vi "Focus Move Absolute.vi"(8 "error in (no error)":errorcluster, 9 "Position":i32, 10 "Motor (0:n-1)":i32, 11 "NewFocus in":refnum<class "NewFocus.lvclass">) -> (0 "error out":errorcluster, 3 "NewFocus out":refnum<class "NewFocus.lvclass">)   [LabVIEW 2021, in "NewFocus.lvclass"]
uses:
  NewFocus.lvclass
  NewFocus.lvclass/NewFocus.ctl
  Focus Class/Focus Class.lvclass
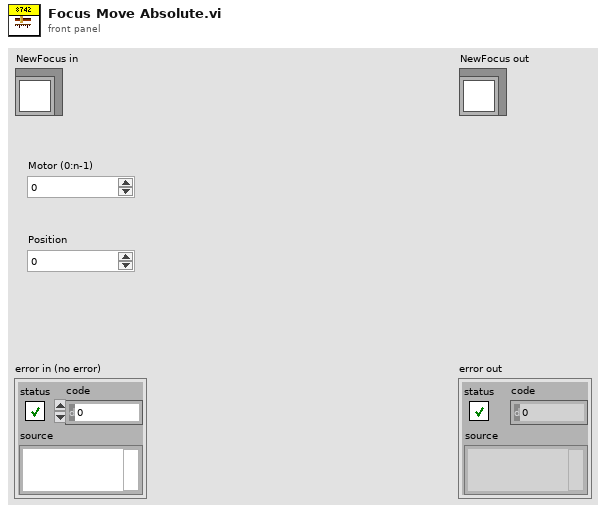
[diagram p1: front panel]
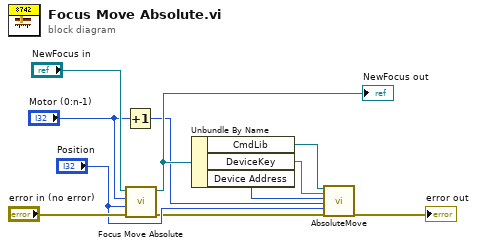
[diagram p0: block diagram]
diagram:
  n1 = Increment(x="Motor (0:n-1)") -> (x+1=w1:i32)
  n2 = call-parent "Focus Move Absolute.vi"("error in (no error)"="error in (no error)", "Position"="Position", "Motor (0:n-1)"="Motor (0:n-1)", "Focus Class in"="NewFocus in") -> ("error out"=w4:errorcluster, "Focus Class out"=w2:refnum<class "NewFocus.lvclass">)  [unwired: 6 in]
  "NewFocus out" <- w2
  n3 = Unbundle By Name(w2) -> ("CmdLib"=w9:refnum<k24>, "DeviceKey"=w8:string, "Device Address"=w7:i32)
  n4 = call "AbsoluteMove.vi"("CmdLib In"=w9, "DeviceKey In"=w8, "Device Address In"=w7, "Motor"=w1, "Target Pos"="Position", "error in (no error)"=w4) -> ("error out"=→"error out":errorcluster)  [unwired: 10 in, 3 out]
